vi "Vision Processing.vi"(4 "error in (no error)":errorcluster, 7 "Image Size":T4=enum."320x240") -> ()   [LabVIEW 2016]
doc: "This VI runs in parallel to other tasks. It gets images from the camera, processes them for color or shape and use that information to affect robot behavior."
uses:
  <vilib>/Rock Robotics/WPI/Camera/WPI_CameraImageSize.ctl
  <vilib>/Rock Robotics/WPI/Camera/WPI_CameraWhite Balance Values.ctl
  <vilib>/Rock Robotics/WPI/Camera/WPI_CameraExposure Values.ctl
  <vilib>/Rock Robotics/WPI/Camera/WPI_CameraFrameRate.ctl
  Google Drive/HowdyBots-Share/BotStuff/2017_SteamWorks/Code/BotCode/Active/Robot Global Data.vi
  <vilib>/Rock Robotics/Network Tables/NT Read Number.vi
  <vilib>/vision/NI_Vision_Development_Module.lvlib
panel:
  in  "Operation":T1(ring)=enum."Erode"
  out "x/y 2":dbl
  in  "Pixel Measurements":T2[](array[typedef])=[35, 4, 5, 6, 7] items=["Center of Mass X", "Center of Mass Y", "First Pixel X", "First Pixel Y", "Bounding Rect Left", "Bounding Rect Top", "Bounding Rect Right", "Bounding Rect Bottom", "Max Feret Diameter Start X", "Max Feret Diameter Start Y", "Max Feret Diameter End X", "Max Feret Diameter End Y", "Max Horiz. Segment Length Left", "Max Horiz. Segment Length Right", "Max Horiz. Segment Length Row", "-", "Bounding Rect Width", "Bounding Rect Height", "Bounding Rect Diagonal", "Perimeter", "Convex Hull Perimeter", "Holes' Perimeter", "Max Feret Diameter", "Equivalent Ellipse Major Axis", "Equivalent Ellipse Minor Axis", "Equivalent Ellipse Minor Axis (Feret)", "Equivalent Rect Long Side", "Equivalent Rect Short Side", "Equivalent Rect Diagonal", "Equivalent Rect Short Side (Feret)", "Average Horiz. Segment Length", "Average Vert. Segment Length", "Hydraulic Radius", "Waddel Disk Diameter", "-", "Area", "Holes' Area", "Particle & Holes' Area", "Convex Hull Area", "Image Area", "-", "Number of Holes", "Number of Horiz. Segments", "Number of Vert. Segments", "-", "Orientation", "Max Feret Diameter Orientation", "-", "% Area/Image Area", "% Area/(Particle & Holes' Area)", "Ratio of Equivalent Ellipse Axes", "Ratio of Equivalent Rect Sides", "-", "Elongation Factor", "Compactness Factor", "Heywood Circularity Factor", "Type Factor", "-", "Sum X", "Sum Y", "Sum XX", "Sum XY", "Sum YY", "Sum XXX", "Sum XXY", "Sum XYY", "Sum YYY", "-", "Moment of Inertia XX", "Moment of Inertia XY", "Moment of Inertia YY", "Moment of Inertia XXX", "Moment of Inertia XXY", "Moment of Inertia XYY", "Moment of Inertia YYY", "Norm. Moment of Inertia XX", "Norm. Moment of Inertia XY", "Norm. Moment of Inertia YY", "Norm. Moment of Inertia XXX", "Norm. Moment of Inertia XXY", "Norm. Moment of Inertia XYY", "Norm. Moment of Inertia YYY", "Hu Moment 1", "Hu Moment 2", "Hu Moment 3", "Hu Moment 4", "Hu Moment 5", "Hu Moment 6", "Hu Moment 7"]
  out "Particles":i32
  in  "Particle Count Limit":dbl=2.0
  out "Min Area Size %":dbl=20.0
  in  "Range":cluster{"Lower value":sgl, "Upper value":sgl}={"Lower value"=241.0, "Upper value"=255.0} {"Upper value" format="%.2f"; "Lower value" format="%.2f"}
  out "Image 2":T3(plugin-control)
  out "Image":T3(plugin-control)
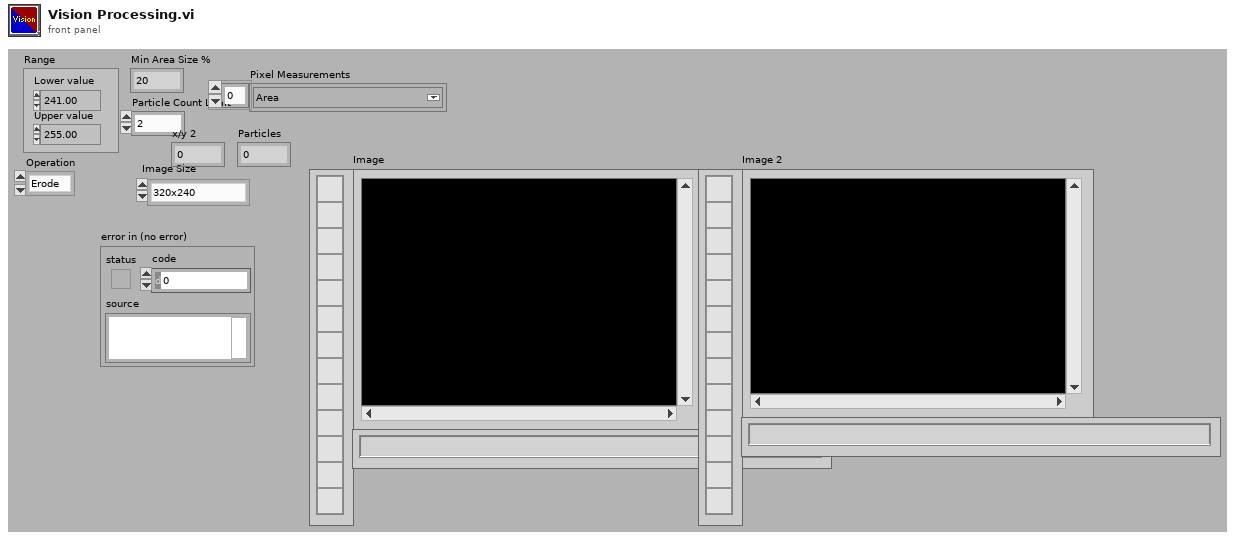
[diagram p1: front panel]
types:
  T1 = enum32{"AutoM", "Close", "Dilate", "Erode", "Gradient", "Gradient in", "Gradient out", "HitMiss", "Open", "PClose", "POpen", "Thick", "Thin"}
  T2 = typedef "Particle Parameters" = i32
  T3 = typedef "IMAQ Image.ctl" = refnum<image>
  T4 = typedef "WPI_CameraImageSize.ctl" = enum16{"640x480", "320x240", "160x120", "Custom"}
  T5 = typedef "Image Type" = u32
  T6 = typedef "WPI_CameraFrameRate.ctl" = u32
  T7 = typedef "WPI_CameraExposure Values.ctl" = enum16{"Auto", "Flicker-free 50 Hz", "Flicker-free 60 Hz", "Hold current", "Custom"}
  T8 = typedef "WPI_CameraWhite Balance Values.ctl" = enum16{"Auto", "Fixed indoor", "Fixed outdoor 1", "Fixed outdoor 2", "Fixed fluorescent 1", "Fixed fluorescent 2", "Hold current", "Custom"}
  T9 = typedef "WPI_CameraDevRef.ctl" = cluster{"Camera Address":string, "CameraStatus":errorcluster}
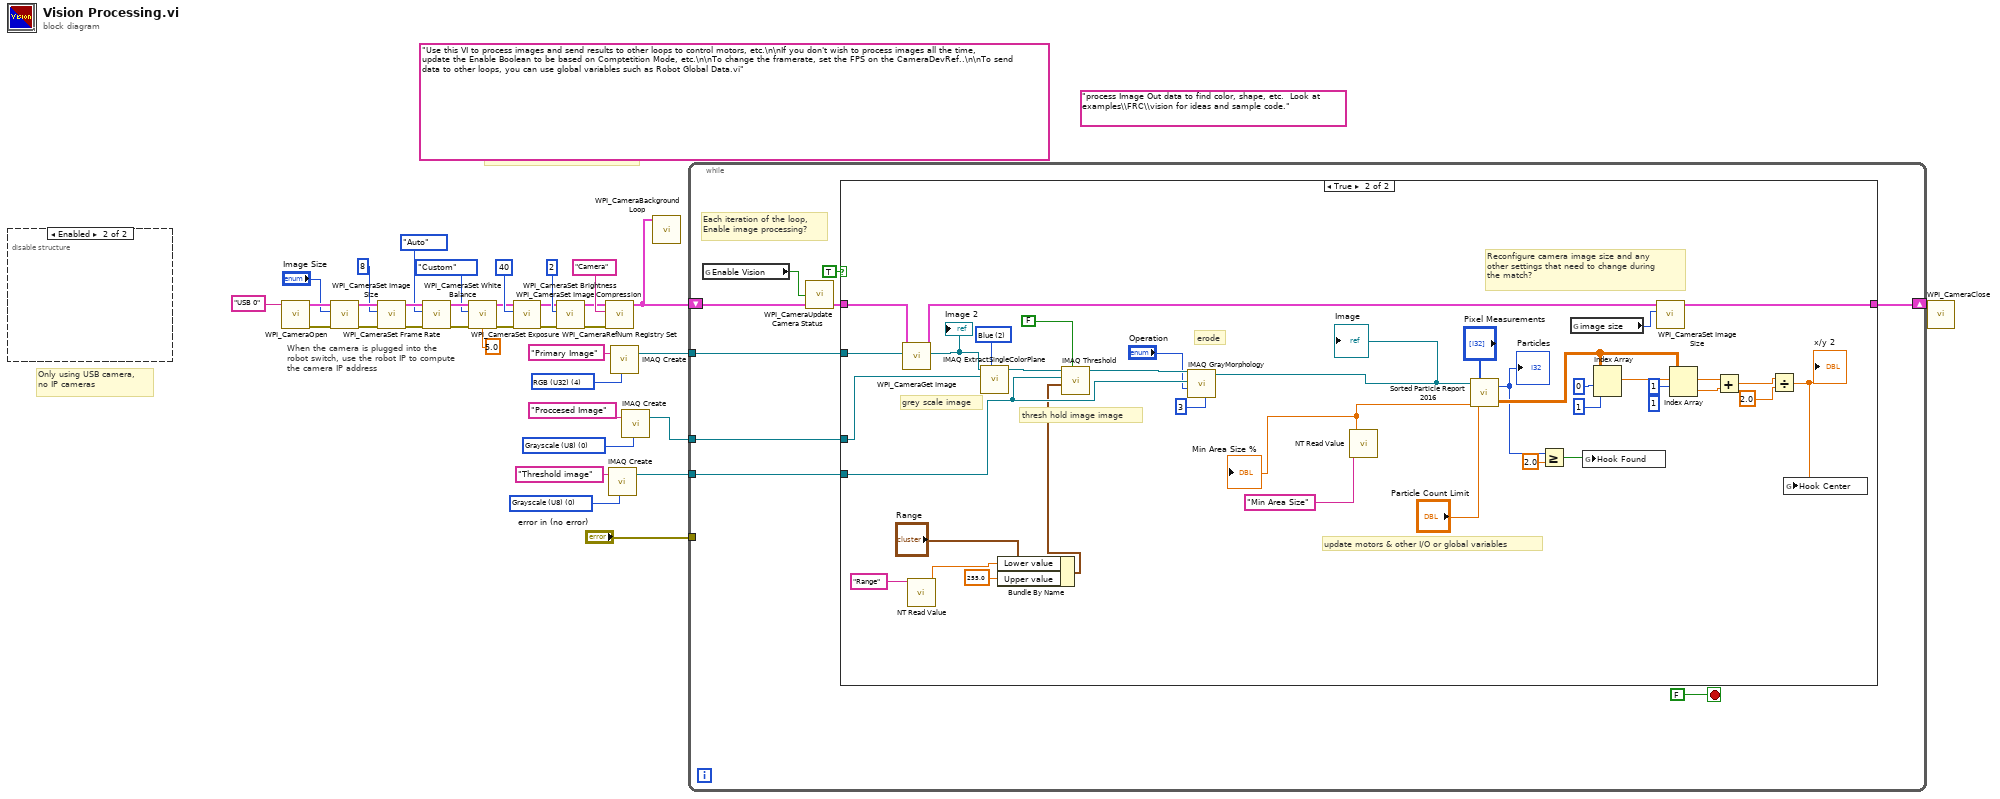
[diagram p0: block diagram]
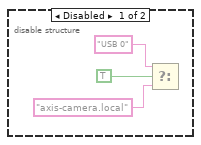
[diagram p2: hidden frame]
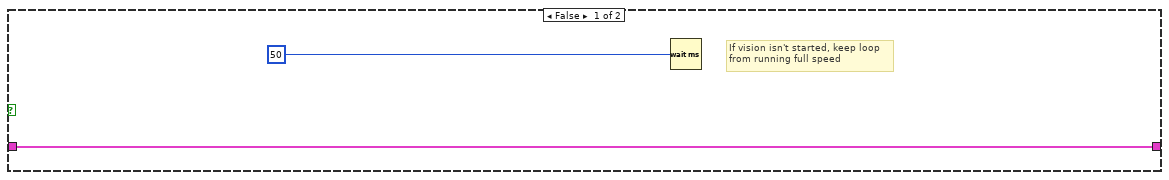
[diagram p3: hidden frame]
diagram:
  (unwired) "process Image Out data to find color, shape, etc.  Look at examples\\FRC\\vision for ideas and sample code."
  w4 = T5 0 items=["Grayscale (U8)", "Grayscale (I16)", "Grayscale (SGL)", "Complex (CSG)", "RGB (U32)", "HSL (U32)", "RGB (U64)"] ("Image Type")
  w7 = T5 0 items=["Grayscale (U8)", "Grayscale (I16)", "Grayscale (SGL)", "Complex (CSG)", "RGB (U32)", "HSL (U32)", "RGB (U64)"] ("Image Type")
  (unwired) "Use this VI to process images and send results to other loops to control motors, etc.\n\nIf you don't wish to process images all the time, update the Enable Boolean to be based on Comptetition Mode, etc.\n\nTo change the framerate, set the FPS on the CameraDevRef..\n\nTo send data to other loops, you can use global variables such as Robot Global Data.vi"
  w35 = T5 4 items=["Grayscale (U8)", "Grayscale (I16)", "Grayscale (SGL)", "Complex (CSG)", "RGB (U32)", "HSL (U32)", "RGB (U64)"] ("Image Type")
  # "Only using USB camera,\nno IP cameras"
  # "When the camera is plugged into the\nrobot switch, use the robot IP to compute\nthe camera IP address"
  # "For Axis cameras, this reads\nimages continuously to avoid\nlatency. For USB, it optionally\nforwards compressed images to\nthe dashboard process."
  n1 = disable-structure shown="Enabled" {
    frame Disabled {
      n2 = Select(t="USB 0" ("format string"), s=TRUE ("dot notation? (F)"), f="axis-camera.local" ("format string")) -> ()  [unwired: 1 out]
    }
    frame Enabled {
    }
  }
  n3 = call <vilib>:"WPI_CameraOpen.vi"("Camera Address"="USB 0" ("format string")) -> ("error out"=w23:errorcluster, "CameraDevRef"=w24:T9)  [unwired: 1 in, 8 out]
  n4 = call <vilib>:"WPI_CameraSet Image Size.vi"("error in (no error)"=w23, "Image Size"="Image Size", "CameraDevRef"=w24) -> ("error out"=w22:errorcluster, "CameraDevRef Out"=w25:T9)  [unwired: 1 in, 6 out]
  n5 = call <vilib>:"WPI_CameraSet Frame Rate.vi"("error in (no error)"=w22, "Frame Rate (fps)"=T6 8, "CameraDevRef"=w25) -> ("error out"=w21:errorcluster, "CameraDevRef Out"=w27:T9)  [unwired: 7 out]
  n6 = call <vilib>:"WPI_CameraSet White Balance.vi"("error in (no error)"=w21, "White Balance"=WPI_CameraWhite_Balance_Values."Auto", "CameraDevRef"=w27) -> ("error out"=w20:errorcluster, "CameraDevRef Out"=w26:T9)  [unwired: 1 in, 6 out]
  n7 = call <vilib>:"WPI_CameraSet Exposure.vi"("error in (no error)"=w20, "Exposure (%)"=5.0, "Exposure"=WPI_CameraExposure_Values."Custom", "CameraDevRef"=w26) -> ("error out"=w19:errorcluster, "CameraDevRef Out"=w29:T9)  [unwired: 6 out]
  n8 = call <vilib>:"WPI_CameraSet Image Compression.vi"("error in (no error)"=w19, "Compression"=40, "CameraDevRef"=w29) -> ("error out"=w18:errorcluster, "CameraDevRef Out"=w28:T9)  [unwired: 7 out]
  n9 = call <vilib>:"WPI_CameraSet Brightness.vi"("error in (no error)"=w18, "Brightness"=2, "CameraDevRef"=w28) -> ("error out"=w16:errorcluster, "CameraDevRef Out"=w17:T9)  [unwired: 7 out]
  n10 = call <vilib>:"WPI_CameraRefNum Registry Set.vi"("error in (no error)"=w16, "refnum name"="Camera", "CameraDevRef"=w17) -> ("CameraDevRef"=w12:T9)  [unwired: 1 in, 7 out]
  n11 = call "IMAQ Create"("Image Name"="Threshold image", "Image Type"=w4) -> ("New Image"=w3:T3)  [unwired: 2 in, 2 out]
  n12 = call "IMAQ Create"("Image Name"="Primary Image", "Image Type"=w35) -> ("New Image"=w33:T3)  [unwired: 2 in, 2 out]
  n13 = call "IMAQ Create"("Image Name"="Proccesed Image", "Image Type"=w7) -> ("New Image"=w6:T3)  [unwired: 2 in, 2 out]
  n14 = call <vilib>:"WPI_CameraBackground Loop.vi"("CameraDevRef"=w12) -> ()  [unwired: 11 in]
  n15 = while {
    shift-right: [w46] -> w10
    shift-left: w12 -> [w44]
    tunnel: w33 -> [w45]
    tunnel: "error in (no error)" -> [_]
    tunnel: w6 -> [w41]
    tunnel: w3 -> [w39]
    stop <- FALSE stop-if-true
    # "Each iteration of the loop,\nEnable image processing?"
    n16 = global read "Robot Global Data.vi" "Enable Vision"() -> (w42:bool)
    n17 = call <vilib>:"WPI_CameraUpdate Camera Status.vi"("CameraDevRef In"=w44, "Enable Vision"=w42) -> ("CameraDevRef Out"=w43:T9)  [unwired: 3 in]
    n18 = case shown="True" TRUE {
      tunnel: w45 -> [_ w85]
      tunnel: [w49 w86] -> w46
      tunnel: w43 -> [w49 w83]
      tunnel: w41 -> [_ w80]
      tunnel: w39 -> [_ w61]
      frame False {
        # "If vision isn't started, keep loop\nfrom running full speed"
        n19 = Wait (ms)(milliseconds to wait=u32 50) -> ()  [unwired: 1 out]
      }
      frame True {
        w50 = 2 items=["Red", "Green", "Blue", "Hue", "Saturation", "Luminance", "Value", "Intensity"] ("Color Plane")
        # "erode"
        # "thresh hold image image"
        # "grey scale image"
        # "update motors & other I/O or global variables"
        # "Reconfigure camera image size and any\nother settings that need to change during\nthe match?"
        n20 = call <vilib>:"WPI_CameraGet Image.vi"("Image"=w85, "CameraDevRef"=w83) -> ("Image Out"=w81:T3, "CameraDevRef Out"=w82:T9)  [unwired: 1 in, 7 out]
        "Image 2" <- w81
        n21 = call-poly <vilib>:"NT Read Value.vi"("Name"="Range") -> ("Numeric"=w58:dbl)  [unwired: 9 in, 1 out]
        n22 = call "IMAQ ExtractSingleColorPlane"("Color Plane"=w50, "Image Dst"=w80, "Image Src"=w81) -> ("Image Dst Out"=w79:T3)  [unwired: 7 in, 1 out]
        n23 = Bundle By Name(cluster="Range", "Lower value"=w58, "Upper value"=sgl 255.0) -> (w56:cluster{"Lower value":sgl, "Upper value":sgl})
        n24 = call "IMAQ Threshold"("Keep/Replace Value (Replace)"=FALSE, "Range"=w56, "Image Dst"=w61, "Image Src"=w79) -> ("Image Dst Out"=w62:T3)  [unwired: 6 in, 1 out]
        n25 = call "IMAQ GrayMorphology"("Number of iterations (1)"=3, "Operation"="Operation", "Image Dst"=w61, "Image Src"=w62) -> ("Image Dst Out"=w60:T3)  [unwired: 6 in, 1 out]
        "Image" <- w60
        n26 = call-poly <vilib>:"NT Read Value.vi"("Name"="Min Area Size") -> ("Numeric"=w54:dbl)  [unwired: 9 in, 1 out]
        "Min Area Size %" <- w54
        n27 = call "Sorted Particle Report 2016.vi"("Min Area Size %"=w54, "Particle Count Limit"="Particle Count Limit", "Pixel Measurements"="Pixel Measurements", "Image in"=w60) -> ("Sorted Data"=w69:dbl[][], "Particles"=w65:i32)
        "Particles" <- w65
        n28 = Greater Or Equal?(x=w65, y=2.0) -> (x >= y?=w64:bool)
        n29 = global read "Robot Global Data.vi" "image size"() -> (w84:T4)
        n30 = global write "Robot Global Data.vi" "Hook Found"(w64) -> ()
        n31 = Index Array(array=w69, index (row)=0, index (col)=1 ("disabled index (col)")) -> (element=w67:dbl)
        n32 = call <vilib>:"WPI_CameraSet Image Size.vi"("Image Size"=w84, "CameraDevRef"=w82) -> ("CameraDevRef Out"=w86:T9)  [unwired: 2 in, 7 out]
        n33 = Index Array(array=w69, index (row)=1, index (col)=1 ("disabled index (col)")) -> (element=w68:dbl)
        n34 = Add(x=w67, y=w68) -> (x+y=w74:dbl)
        n35 = Divide(x=w74, y=2.0) -> (x/y=w63:dbl)
        "x/y 2" <- w63
        n36 = global write "Robot Global Data.vi" "Hook Center"(w63) -> ()
      }
    }
  }
  n37 = call <vilib>:"WPI_CameraClose.vi"("CameraDevRef"=w10) -> ()  [unwired: 1 in, 10 out]
